vi "RT Loop - Analyze Acceleration_queue.vi"(7 "testing":bool, 8 "error in (no error)":errorcluster, 9 "Acceleration RT FIFO In":T1, 10 "FPGA VI Reference Out":refnum<k20>, 11 "Message Queue":refnum<queue>) -> (1 "Acceleration RT FIFO Out":T1)   [LabVIEW 2017]
doc: "Read and analyze acceleration waveform data from FPGA via DMA FIFO. If the acceleration is over the limit, then send the acceleration waveform data to the Log Data Loop."
uses:
  UI Error Handlers/support/Message Queue/Message Cluster.ctl
  controls/Acceleration RT FIFO Reference.ctl
  Globals/Global - Configuration Options.vi
  Globals/Global - All RT Loop Stop.vi
  <vilib>/Utility/error.llb/Error Cluster From Error Code.vi
  <vilib>/rvi/errors/niLvFpgaAdjustHostInterfaceError.vi
  <vilib>/rvi/interface/nirviMethod/nirviMethod.xnode
  <vilib>/FPGAPlugInAG/Dynamic/niLvFpga_ReadFifo_Dynamic.vi
  <vilib>/rvi/errors/niLvFpgaMergeErrorWithErrorCode.vi
  UI Error Handlers/support/Logging/Logging.lvlib
  UI Error Handlers/support/Message Queue/Message Queue.lvlib
panel:
  out "error out 2":errorcluster
  out "AVI Path":path
  out "G1 status.G1 trigger 2":bool
  out "error out":errorcluster
  out "Array":waveform(dbl)[](array[waveform])
  out "x-y":u32
  out "G1 status":cluster{"G1 trigger":bool}
  out "G1 status.G1 trigger":bool
  out "sta":bool
  out "logical OR":bool
  in  "Data Rate (Hz)":dbl
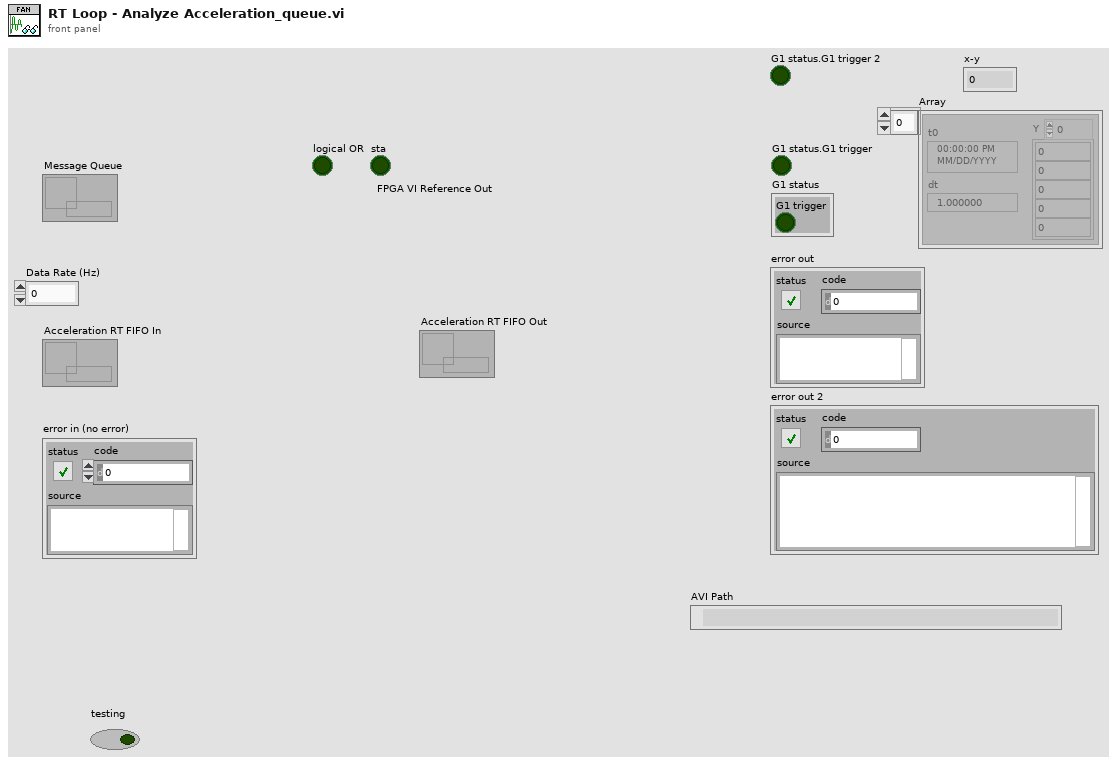
[diagram p1: front panel]
types:
  T1 = typedef "Acceleration RT FIFO Reference.ctl" = refnum<k33>
  T2 = cluster{"Tool data":cluster{"Number of teeth":sgl}, "Cutting data":cluster{"rpm":sgl}, "Limits":cluster{"Magnitude threshold":sgl, "Tolerance":sgl}, "G1 status":cluster{"G1 trigger":bool}}
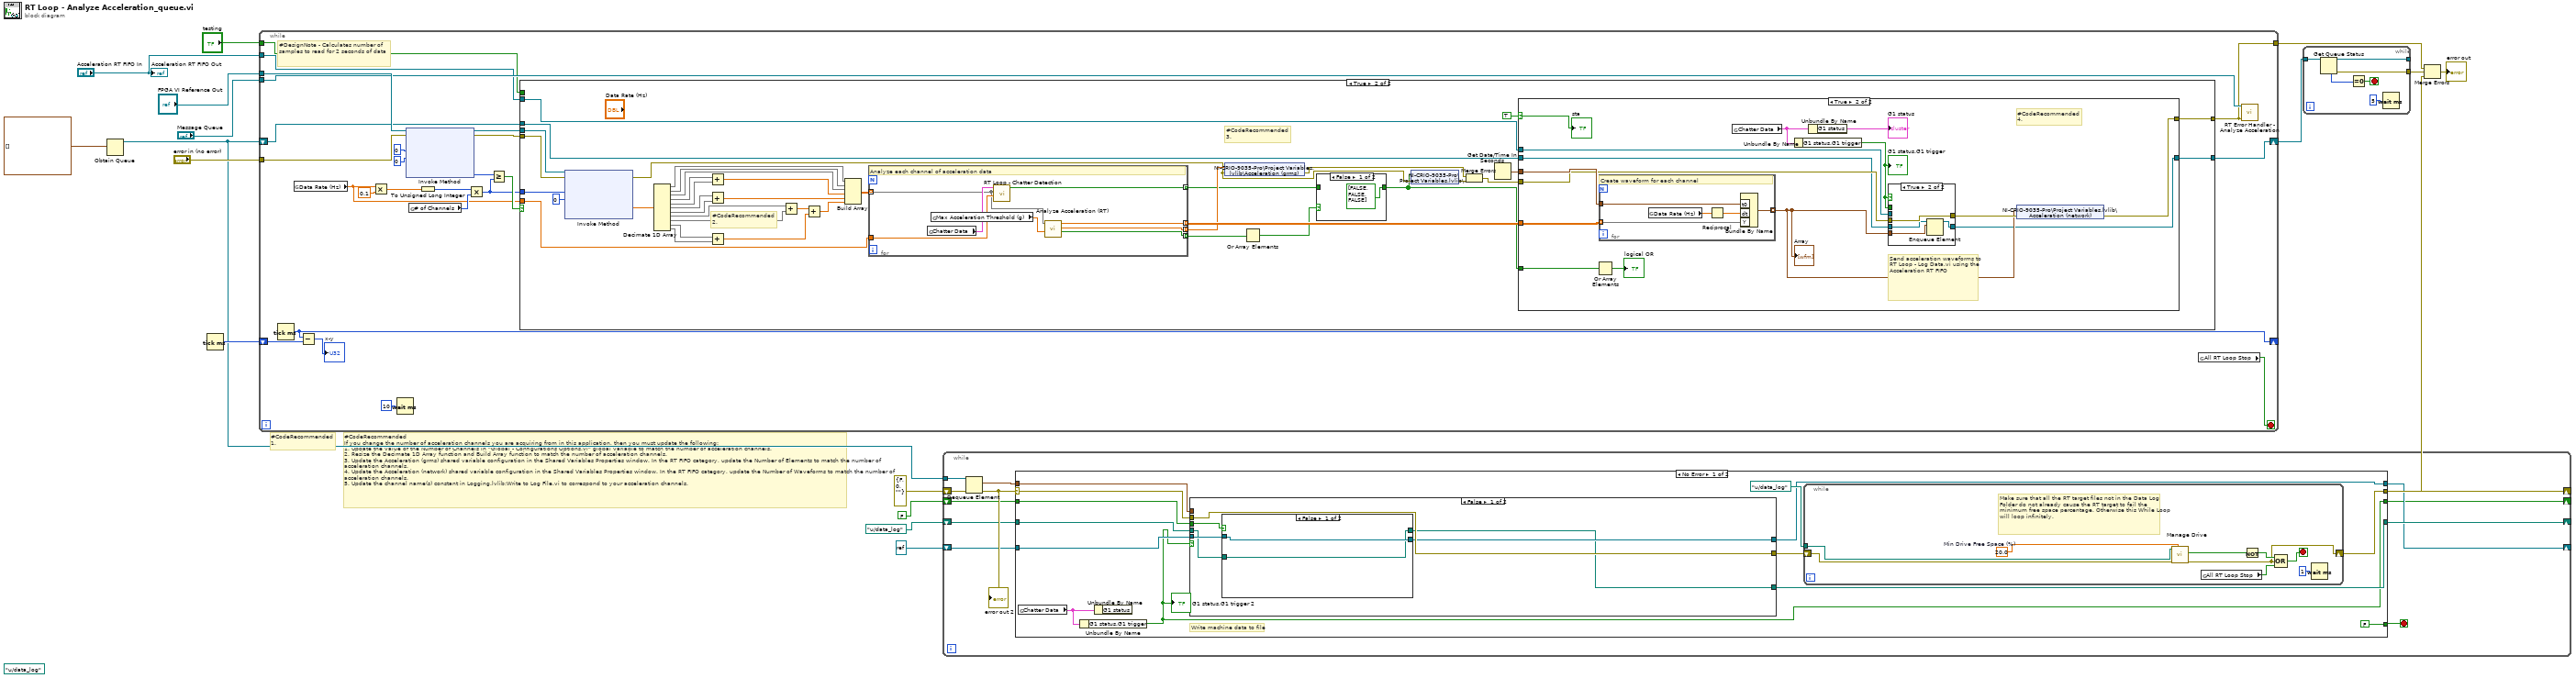
[diagram p0: block diagram]
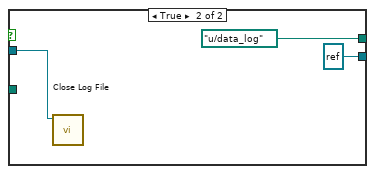
[diagram p2: hidden frame]
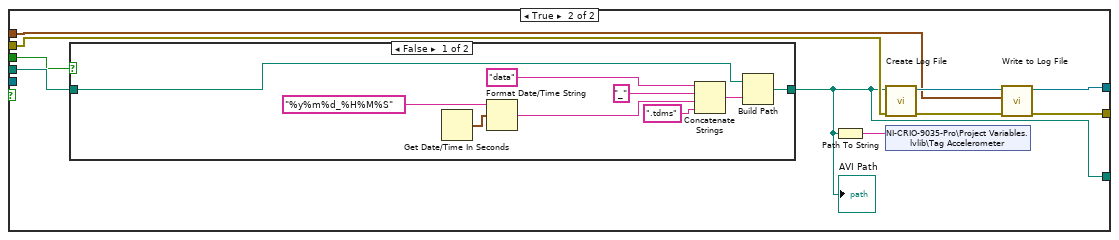
[diagram p3: hidden frame]
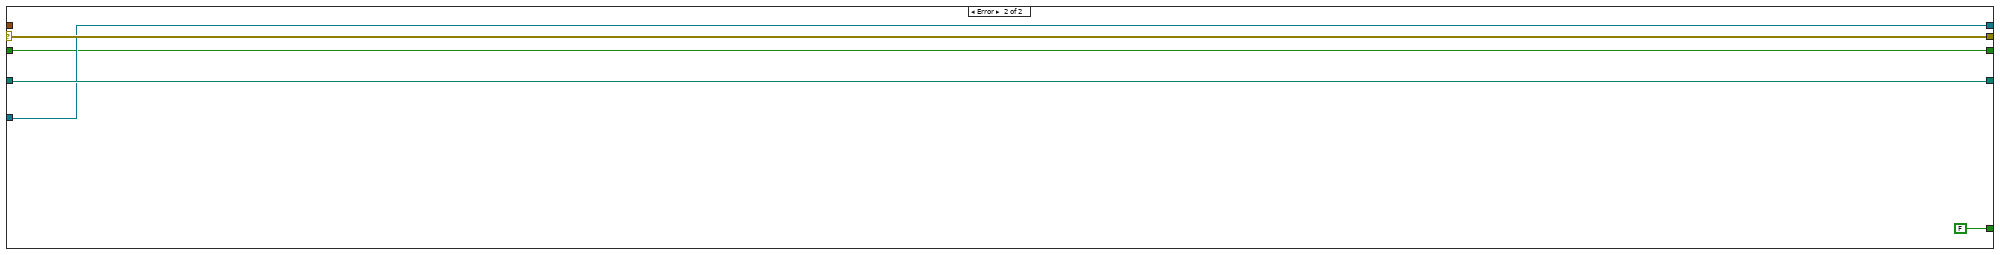
[diagram p5: hidden frame]
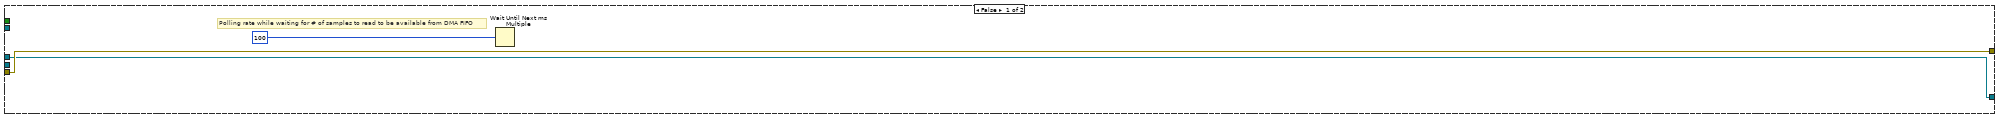
[diagram p6: hidden frame]
diagram:
  (unwired) path "u:/data_log" ("AVI Path")
  # "#CodeRecommended\n1."
  # "#CodeRecommended\nIf you change the number of acceleration channels you are acquiring from in this application, then you must update the following:\n1. Update the value of the Number of Channels in \"Global - Configurations Options.vi\" global variable to match the number of acceleration channels.\n2. Resize the Decimate 1D Array function and Build Array function to match the number of acceleration channels. \n3. Update the Acceleration (grms) shared variable configuration in the Shared Variables Properties window. In the RT FIFO category, update the Number of Elements to match the number of acceleration channels. \n4. Update the Acceleration (network) shared variable configuration in the Shared Variables Properties window. In the RT FIFO category, update the Number of Waveforms to match the number of acceleration channels.\n5. Update the channel name(s) constant in Logging.lvlib:Write to Log File.vi to correspond to your acceleration channels."
  n1 = Obtain Queue(element data type=waveform(dbl)[] [] ("Array 2")) -> (queue out=w5:refnum<queue>)  [unwired: 4 in, 2 out]
  n2 = Tick Count (ms)() -> (millisecond timer value=w12:u32)
  n3 = while {
    tunnel: "FPGA VI Reference Out" -> [w42]
    tunnel: "error in (no error)" -> [w41]
    tunnel: "Message Queue" -> [w34]
    tunnel: "Acceleration RT FIFO In" -> [w33]
    tunnel: "testing" -> [w25]
    shift-right: [w23] -> _
    shift-left: w12 -> [w24]
    shift-right: [w20] -> w4
    shift-left: w5 -> [w21]
    tunnel: [w19] -> w2
    stop <- w35 stop-if-true
    # "#DesignNote - Calculates number of samples to read for 2 seconds of data"
    n4 = Tick Count (ms)() -> (millisecond timer value=w23:u32)
    n5 = global read "Global - Configuration Options.vi" "Data Rate (Hz)"() -> (w27:dbl)
    n6 = Subtract(x=w23, y=w24) -> (x-y=→"x-y":u32)
    n7 = Multiply(x=w27, y=0.1) -> (x*y=w31:dbl)
    n8 = Wait (ms)(milliseconds to wait=u32 10) -> ()  [unwired: 1 out]
    n9 = xnode "Invoke Method"("FPGA VI Reference In"=w42, "error in"=w41, "Number of Elements"=u32 0, "Timeout (ms)"=0) -> ("FPGA VI Reference Out"=w38:refnum<k20>, "error out"=w37:errorcluster, "Elements Remaining"=w26:u32)  [unwired: 1 out]
    n10 = global read "Global - Configuration Options.vi" "# of Channels"() -> (w28:u32)
    n11 = To Unsigned Long Integer(number=w31) -> (unsigned 32bit integer=w30:u32)
    n12 = Multiply(x=w30, y=w28) -> (x*y=w29:u32)
    n13 = Greater Or Equal?(x=w26, y=w29) -> (x >= y?=w36:bool)
    n14 = case shown="True" w36 {
      tunnel: w38 -> [_ w84]
      tunnel: w37 -> [w45 w83]
      tunnel: [w45 w79] -> w19
      tunnel: w29 -> [_ w82]
      tunnel: w33 -> [_ w77]
      tunnel: w27 -> [_ w73]
      tunnel: w25 -> [_ _]
      tunnel: w21 -> [w43 w47]
      tunnel: [w43 w46] -> w20
      frame False {
        # "Polling rate while waiting for # of samples to read to be available from DMA FIFO"
        n15 = Wait Until Next ms Multiple(millisecond multiple=u32 100) -> ()  [unwired: 1 out]
      }
      frame True {
        # "#CodeRecommended\n3."
        # "#CodeRecommended\n2."
        n16 = xnode "Invoke Method"("FPGA VI Reference In"=w84, "error in"=w83, "Number of Elements"=w82, "Timeout (ms)"=0) -> ("error out"=w72:errorcluster, "Data"=w76:sgl[])  [unwired: 2 out]
        n17 = Decimate 1D Array(w76) -> (w63:sgl[], w62:sgl[], w61:sgl[], w60:sgl[], w59:sgl[], w57:sgl[], w56:sgl[], w55:sgl[], w54:sgl[], w53:sgl[], w52:sgl[])
        n18 = Add(x=w60, y=w59) -> (x+y=w58:sgl[])
        n19 = Add(x=w57, y=w56) -> (x+y=w48:sgl[])
        n20 = Add(x=w53, y=w52) -> (x+y=w50:sgl[])
        n21 = Add(x=w55, y=w54) -> (x+y=w51:sgl[])
        n22 = Add(x=w51, y=w50) -> (x+y=w49:sgl[])
        n23 = Build Array(w63, w62, w61, w58, w48, w49) -> (w64:sgl[][])
        n24 = for {
          tunnel: [w94] -> w78 mode=indexing
          tunnel: [w93] -> w75 mode=indexing
          tunnel: [w92] -> w74 mode=indexing
          tunnel: w73 -> [w90]
          tunnel: [w89] -> w67 mode=indexing
          tunnel: w64 -> [w87] mode=indexing
          # "Analyze each channel of acceleration data"
          n25 = global read "Global - Configuration Options.vi" "Chatter Data"() -> (w88:T2)
          n26 = global read "Global - Configuration Options.vi" "Max Acceleration Threshold (g)"() -> (w91:sgl)
          n27 = call "RT Loop - Chatter Detection.vi"("Data Rate (Hz)"=w90, "Acceleration Waveform (SGL)"=w87, "Chatter Data"=w88) -> ("Chatter?"=w89:bool)  [unwired: 8 in]
          n28 = call "Analyze Acceleration (RT).vi"("Max Instantaneous Acceleration (g)"=w91, "Acceleration Waveform (SGL)"=w87) -> ("Over Limit?"=w94:bool, "Acceleration (grms)"=w92:dbl, "Acceleration Waveform (DBL)"=w93:dbl[])  [unwired: 7 in]
        }
        n29 = shared-variable "NI-CRIO-9035-Pro\\Project Variables.lvlib\\Acceleration (grms)"(w74, error in=w72) -> (error out=w70:errorcluster)
        n30 = Or Array Elements(Boolean array=w78) -> (logical OR=w68:bool)
        n31 = case shown="False" w68 {
          tunnel: w67 -> [_ w86]
          tunnel: [bool[] [FALSE, FALSE, FALSE] ("Chatter?") w86] -> w66
          frame False {
          }
          frame True {
          }
        }
        n32 = shared-variable "NI-CRIO-9035-Pro\\Project Variables.lvlib\\Chatter?"(w66, error in=w72) -> (error out=w71:errorcluster)
        n33 = Merge Errors(w70, w71) -> (w69:errorcluster)
        n34 = Get Date/Time In Seconds() -> (seconds since 1Jan1904=w80:timestamp)
        n35 = case shown="True" TRUE {
          selector: TRUE -> [_ w104]
          tunnel: w80 -> [_ w111]
          tunnel: w69 -> [w96 w110]
          tunnel: [w96 w109] -> w79
          tunnel: w77 -> [_ w108]
          tunnel: w75 -> [_ w107]
          tunnel: w66 -> [_ w105]
          tunnel: w47 -> [w95 w98]
          tunnel: [w95 w97] -> w46
          frame False {
          }
          frame True {
            # "#CodeRecommended\n4."
            # "Send acceleration waveforms to RT Loop - Log Data.vi using the Acceleration RT FIFO"
            n36 = Or Array Elements(Boolean array=w105) -> (logical OR=→"logical OR":bool)
            n37 = for {
              tunnel: w107 -> [w122] mode=indexing
              tunnel: w111 -> [w121]
              tunnel: [w119] -> w99 mode=indexing
              # "Create waveform for each channel"
              n38 = global read "Global - Configuration Options.vi" "Data Rate (Hz)"() -> (w118:dbl)
              n39 = Reciprocal(x=w118) -> (1/x=w120:dbl)
              n40 = Bundle By Name("t0"=w121, "dt"=w120, "Y"=w122) -> (w119:waveform(dbl))  [unwired: 1 in]
            }
            "Array" <- w99
            n41 = global read "Global - Configuration Options.vi" "Chatter Data"() -> (w103:T2)
            n42 = Unbundle By Name(w103) -> ("G1 status.G1 trigger"=w100:bool)
            "G1 status.G1 trigger" <- w100
            n43 = Unbundle By Name(w103) -> ("G1 status"=→"G1 status":cluster{"G1 trigger":bool})
            n44 = case shown="True" w100 {
              tunnel: w110 -> [w113 w117]
              tunnel: w99 -> [_ w114]
              tunnel: w108 -> [_ _]
              tunnel: w100 -> [_ _]
              tunnel: [w113 w117] -> w101
              tunnel: w98 -> [w112 w116]
              tunnel: [w112 w115] -> w97
              frame False {
              }
              frame True {
                n45 = Enqueue Element(queue=w116, element=w114) -> (queue out=w115:refnum<queue>)  [unwired: 2 in, 2 out]
              }
            }
            n46 = shared-variable "NI-CRIO-9035-Pro\\Project Variables.lvlib\\Acceleration (network)"(w99, error in=w101) -> (error out=w109:errorcluster)
            "sta" <- w104
          }
        }
      }
    }
    n47 = global read "Global - All RT Loop Stop.vi" "All RT Loop Stop"() -> (w35:bool)
    n48 = call "RT Error Handler - Analyze Acceleration.vi"("error in (no error)"=w19, "Message Queue"=w34) -> ()  [unwired: 9 in, 1 out]
  }
  n49 = while {
    tunnel: w5 -> [w134]
    shift-right: [w130] -> w8
    shift-left: errorcluster {"status"=FALSE, "code"=0, "source"=""} ("error in (no error)") -> [w133]
    shift-right: [w123] -> _
    shift-left: FALSE ("Boolean") -> [w126]
    shift-right: [w128] -> _
    shift-left: path "u:/data_log" ("AVI Path") -> [w129]
    shift-right: [w125] -> _
    shift-left: refnum<k34> refnum ("Log File out") -> [w124]
    stop <- w131 stop-if-true
    n50 = Dequeue Element(queue=w134, error in (no error)=w133) -> (element=w127:waveform(dbl)[], error out=w132:errorcluster)  [unwired: 1 in, 2 out]
    "error out 2" <- w132
    n51 = case shown="No Error" w132 {
      selector: w132 -> [w142 w191]
      tunnel: [FALSE FALSE] -> w131
      tunnel: [w140 w191] -> w130
      tunnel: w129 -> [w146 w190]
      tunnel: [w145 w190] -> w128
      tunnel: w127 -> [w144 _]
      tunnel: w126 -> [w139 w188]
      tunnel: [w138 w189] -> w125
      tunnel: w124 -> [w137 w189]
      tunnel: [w135 w188] -> w123
      frame No Error {
        # "Write machine data to file"
        n52 = global read "Global - Configuration Options.vi" "Chatter Data"() -> (w136:T2)
        n53 = Unbundle By Name(w136) -> ("G1 status.G1 trigger"=w135:bool)
        "G1 status.G1 trigger 2" <- w135
        n54 = Unbundle By Name(w136) -> ()  [unwired: 1 out]
        n55 = case shown="False" w135 {
          tunnel: w146 -> [w157 w177]
          tunnel: [w158 w169] -> w145
          tunnel: w144 -> [_ w173]
          tunnel: w142 -> [w162 w172]
          tunnel: [w162 w171] -> w141
          tunnel: w139 -> [w161 w168]
          tunnel: [w159 w170] -> w138
          tunnel: w137 -> [w160 _]
          frame False {
            n56 = case shown="False" w161 {
              tunnel: [w163 path "u:/data_log" ("AVI Path")] -> w158
              tunnel: w160 -> [w164 w166]
              tunnel: [w164 refnum<k34> refnum ("Log File out")] -> w159
              tunnel: w157 -> [w163 _]
              frame False {
              }
              frame True {
                n57 = call "Close Log File.vi"("tdms file"=w166) -> ()  [unwired: 10 in, 1 out]
              }
            }
          }
          frame True {
            n58 = case shown="False" w168 {
              tunnel: w177 -> [w180 w187]
              tunnel: [w179 w187] -> w169
              frame False {
                n59 = Get Date/Time In Seconds() -> (seconds since 1Jan1904=w182:timestamp)
                n60 = Format Date/Time String(time format string (%c)="%y%m%d_%H%M%S", seconds (now)=w182) -> (date/time string=w185:string)  [unwired: 1 out]
                n61 = Concatenate Strings("data" ("string"), "_" ("string"), w185, ".tdms" ("string")) -> (w181:string)
                n62 = Build Path(base path=w180, name or relative path=w181) -> (appended path=w179:path)
              }
              frame True {
              }
            }
            "AVI Path" <- w169
            n63 = Path To String(path=w169) -> (string=w174:string)
            n64 = call "Create Log File.vi"("error in (no error)"=w172, "Acceleration Exceeded Log Folder"=w169) -> ("error out"=w176:errorcluster, "Log File out"=w175:refnum<k34>)  [unwired: 8 in]
            n65 = shared-variable "NI-CRIO-9035-Pro\\Project Variables.lvlib\\Tag Accelerometer"(w174) -> ()  [unwired: 1 in, 1 out]
            n66 = call "Write to Log File.vi"("error in (no error)"=w176, "Array of Waveforms"=w173, "Log File in"=w175) -> ("error out"=w171:errorcluster, "Log File out"=w170:refnum<k34>)  [unwired: 7 in]
          }
        }
        n67 = while {
          shift-right: [w151] -> w140
          shift-left: w141 -> [w152]
          tunnel: path "u:/data_log" ("AVI Path") -> [w149]
          stop <- w156 stop-if-true
          w150 = 20.0  # Min Drive Free Space (%)
          # "Make sure that all the RT target files not in the Data Log Folder do not already cause the RT target to fail the minimum free space percentage. Otherwise this While Loop will loop infinitely."
          n68 = call "Manage Drive.vi"("Min Drive Free Space (%)"=w150, "error in"=w152, "Data Folder"=w149) -> ("error out"=w151:errorcluster, "Drive Space Below Limit"=w148:bool)  [unwired: 7 in]
          n69 = global read "Global - All RT Loop Stop.vi" "All RT Loop Stop"() -> (w153:bool)
          n70 = Not(x=w148) -> (.not. x?=w155:bool)
          n71 = Compound Arithmetic op=OR(w155, w151, w153) -> (w156:bool)
          n72 = Wait (ms)(milliseconds to wait=u32 1) -> ()  [unwired: 1 out]
        }
      }
      frame Error {
      }
    }
  }
  n73 = while {
    tunnel: [w197] -> w3
    tunnel: [w195] -> _
    tunnel: w4 -> [w193]
    stop <- w196 stop-if-true
    n74 = Get Queue Status(queue=w193) -> (queue out=w195:refnum<queue>, error out=w197:errorcluster, # elements in queue=w194:i32)  [unwired: 2 in, 5 out]
    n75 = Equal To 0?(x=w194) -> (x = 0?=w196:bool)
    n76 = Wait (ms)(milliseconds to wait=u32 5) -> ()  [unwired: 1 out]
  }
  n77 = Merge Errors(w2, w3, w8) -> (→"error out":errorcluster)
  "Acceleration RT FIFO Out" <- "Acceleration RT FIFO In"
